vi "pid_main_v2.vi"(5 "limits":T5={"upperLimit"=2.0, "lowerLimit"=0.0}, 6 "ready for output (T)":bool=TRUE, 7 "manualMotion":T1, 8 "inputValid":bool=TRUE, 9 "liftOffParams":T3={"liftHeight"=0.0498046875, "disengagePos"=-1.0, "liftOff"=FALSE} {"disengagePos" format="%#_28g"}, 10 "fbParams":T4={"enable"=FALSE, "setPoint"=0.001007080078125, "pGain"=0.0, "iGain"=0.10000038146972656, "gainScale"=0}, 11 "input":fxp<+/-,24,16>) -> (0 "output valid":bool, 3 "output":T2, 4 "ready for input":bool)   [LabVIEW 2016]
uses:
  <vilib>/rvi/FXPMathLib/FxpAdd/XNode/nifxpmath_Add.xnode
  <vilib>/rvi/FXPMathLib/FxpInterpret/XNode/nifxpmath_Interpret.xnode
  <vilib>/rvi/FXPMathLib/FxpSub/XNode/nifxpmath_Sub.xnode
  <vilib>/rvi/FXPMathLib/FxpMul/XNode/nifxpmath_Multiplier.xnode
  <vilib>/rvi/FXPMathLib/sim/FxpSim.dll
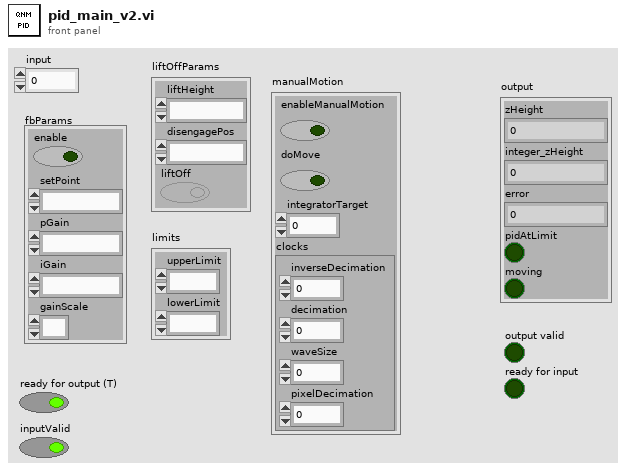
[diagram p1: front panel]
types:
  T1 = cluster{"enableManualMotion":bool, "doMove":bool, "integratorTarget":fxp<+/-,22,2>, "clocks":cluster{"inverseDecimation":fxp<+,22,0>, "decimation":u16, "waveSize":u16, "pixelDecimation":u16}}
  T2 = cluster{"zHeight":fxp<+/-,28,1>, "integer_zHeight":i16, "error":fxp<+/-,25,2>, "pidAtLimit":bool, "moving":bool}
  T3 = cluster{"liftHeight":fxp<+/-,15,4>, "disengagePos":fxp<+/-,22,1>, "liftOff":bool}
  T4 = cluster{"enable":bool, "setPoint":fxp<+/-,17,1>, "pGain":fxp<+/-,20,4>, "iGain":fxp<+/-,20,1>, "gainScale":i8}
  T5 = cluster{"upperLimit":fxp<+/-,28,4>, "lowerLimit":fxp<+/-,28,4>}
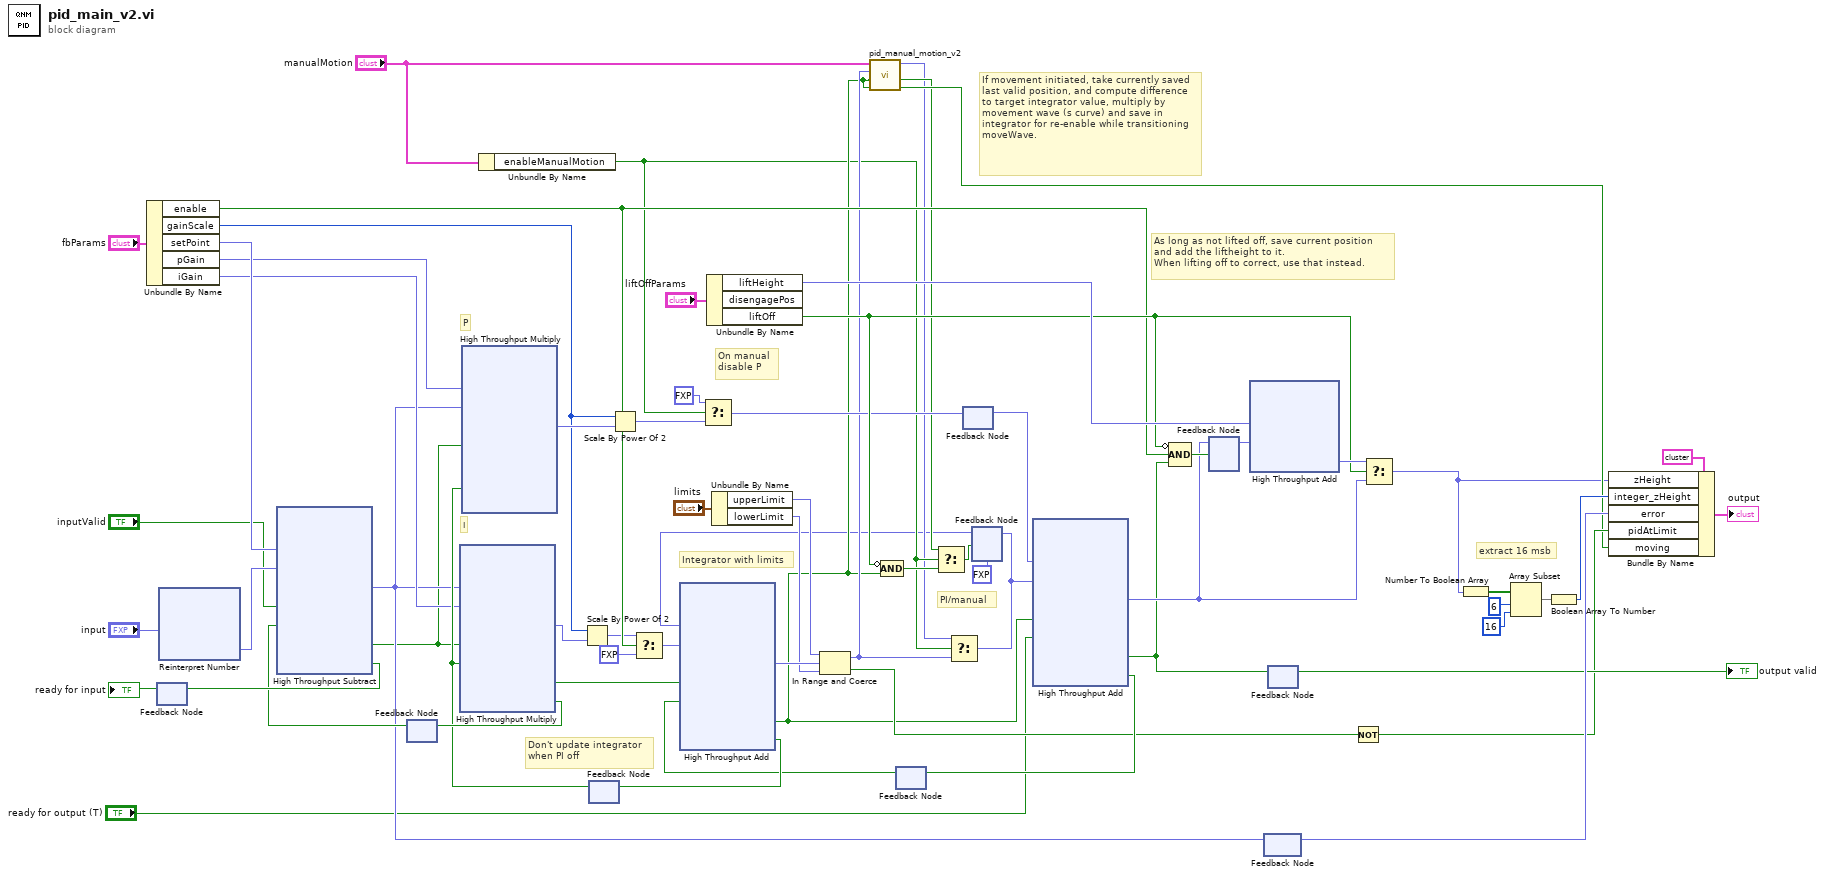
[diagram p0: block diagram]
diagram:
  # "Don't update integrator\nwhen PI off"
  # "On manual\ndisable P"
  # "PI/manual"
  # "I"
  # "P"
  # "If movement initiated, take currently saved last valid position, and compute difference to target integrator value, multiply by movement wave (s curve) and save in integrator for re-enable while transitioning moveWave."
  # "Integrator with limits"
  # "As long as not lifted off, save current position\nand add the liftheight to it.\nWhen lifting off to correct, use that instead."
  # "extract 16 msb"
  n1 = Unbundle By Name("fbParams") -> ("enable"=w30:bool, "gainScale"=w38:i8, "setPoint"=w41:fxp<+/-,17,1>, "pGain"=w40:fxp<+/-,20,4>, "iGain"=w39:fxp<+/-,20,1>)
  n2 = feedback #1() -> (→"ready for input":bool)  [unwired: 1 in]
  n3 = xnode "Reinterpret Number"("x"="input") -> ("y"=w45:fxp<+/-,24,1>)
  n4 = feedback #2() -> (w63:bool)  [unwired: 1 in]
  n5 = xnode ("High Throughput Subtract")("x"=w41, "y"=w45, "input valid"="inputValid", "ready for output (T)"=w63) -> ("x-y"=w32:fxp<+/-,25,2>, "output valid"=w20:bool, "ready for input"=w66:bool)
  n6 = feedback-in #1(w66) -> ()
  n7 = Unbundle By Name("manualMotion") -> ("enableManualMotion"=w13:bool)
  n8 = feedback #3() -> (w59:bool)  [unwired: 1 in]
  n9 = xnode ("High Throughput Multiply")("x"=w32, "y"=w39, "input valid"=w20, "ready for output (T)"=w59) -> ("x*y"=w61:fxp<+/-,32,2>, "output valid"=w58:bool, "ready for input"=w64:bool)
  n10 = feedback-in #2(w64) -> ()
  n11 = xnode ("High Throughput Multiply")("x"=w40, "y"=w32, "input valid"=w20, "ready for output (T)"=w59) -> ("x*y"=w55:fxp<+/-,32,2>)  [unwired: 2 out]
  n12 = Scale By Power Of 2(n=w38, x=w61) -> (x*2^n=w3:fxp<+/-,32,2>)
  n13 = Scale By Power Of 2(n=w38, x=w55) -> (x*2^n=w43:fxp<+/-,32,2>)
  n14 = Select(t=w3, s=w30, f=fxp<+/-,32,2> 0.0) -> (s? t:f=w2:fxp<+/-,32,2>)
  n15 = Select(t=fxp<+/-,32,2> 0.0, s=w13, f=w43) -> (s? t:f=w24:fxp<+/-,32,2>)
  n16 = Unbundle By Name("liftOffParams") -> ("liftHeight"=w35:fxp<+/-,15,4>, "liftOff"=w34:bool)  [unwired: 1 out]
  n17 = Unbundle By Name("limits") -> ("upperLimit"=w56:fxp<+/-,28,4>, "lowerLimit"=w57:fxp<+/-,28,4>)
  n18 = feedback #4() -> (w25:bool)  [unwired: 1 in]
  n19 = feedback #5() -> (w53:fxp<+/-,32,2>)  [unwired: 1 in]
  n20 = feedback-in #5(w24) -> ()
  n21 = feedback #6(fxp<+/-,32,4> -1.0 ("x+y")) -> (w4:fxp<+/-,32,4>)
  n22 = xnode ("High Throughput Add")("x"=w4, "y"=w2, "input valid"=w58, "ready for output (T)"=w25) -> ("x+y"=w62:fxp<+/-,32,4>, "output valid"=w16:bool, "ready for input"=w60:bool)
  n23 = feedback-in #3(w60) -> ()
  n24 = In Range and Coerce(upper limit=w56, x=w62, lower limit=w57) -> (coerced(x)=w17:fxp<+/-,32,4>, In Range?=w27:bool)
  n25 = call "pid_manual_motion_v2.vi"("inputValid"=w16, "lastPosValid"=w16, "lastPos"=w17, "manualMotion"="manualMotion") -> ("moving"=w18:bool, "outputValid"=w12:bool, "output"=w6:fxp<+/-,32,4>)  [unwired: 5 in]
  n26 = Compound Arithmetic op=AND(invert w34, w16) -> (w14:bool)
  n27 = Select(t=w12, s=w13, f=w14) -> (s? t:f=w15:bool)
  n28 = Select(t=w6, s=w13, f=w17) -> (s? t:f=w5:fxp<+/-,32,4>)
  n29 = feedback-in #6(w5, w15) -> ()
  n30 = xnode ("High Throughput Add")("x"=w53, "y"=w5, "input valid"=w16, "ready for output (T)"="ready for output (T)") -> ("x+y"=w10:fxp<+/-,22,1>, "output valid"=w9:bool, "ready for input"=w54:bool)
  n31 = feedback-in #4(w54) -> ()
  n32 = Compound Arithmetic op=AND(invert w34, w30, w9) -> (w49:bool)
  n33 = feedback #7() -> (w47:fxp<+/-,22,1>)  [unwired: 1 in]
  n34 = feedback-in #7(w10, w49) -> ()
  n35 = xnode ("High Throughput Add")("x"=w35, "y"=w47) -> ("x+y"=w46:fxp<+/-,22,1>)
  n36 = feedback #8() -> (w31:fxp<+/-,25,2>)  [unwired: 1 in]
  n37 = feedback-in #8(w32) -> ()
  n38 = feedback #9() -> (→"output valid":bool)  [unwired: 1 in]
  n39 = feedback-in #9(w9) -> ()
  n40 = Not(x=w27) -> (.not. x?=w21:bool)
  n41 = Select(t=w46, s=w34, f=w10) -> (s? t:f=w7:fxp<+/-,22,1>)
  n42 = Number To Boolean Array(number=w7) -> (Boolean array=w50:bool[])
  n43 = Array Subset(array=w50, index=6, length=16) -> (w48:bool[])
  n44 = Boolean Array To Number(Boolean array=w48) -> (number=w33:i16)
  n45 = Bundle By Name(cluster=T2 {"zHeight"=0.0, "integer_zHeight"=0, "error"=0.0, "pidAtLimit"=FALSE, "moving"=FALSE} ("output"), "zHeight"=w7, "integer_zHeight"=w33, "error"=w31, "pidAtLimit"=w21, "moving"=w18) -> (→"output":T2)
